vi "Initialize Device.vi"(8 "error in (no error)":errorcluster, 10 "VISA resource name":refnum<visa-resource-name>="COM9", 11 "Simulated in":refnum<class "Simulated.lvclass">) -> (0 "error out":errorcluster, 3 "Simulated out":refnum<class "Simulated.lvclass">)   [LabVIEW 2019, in "Simulated.lvclass"]
uses:
  Simulated.lvclass
  Abstract Spectrometer_class/Abstract Spectrometer.lvclass
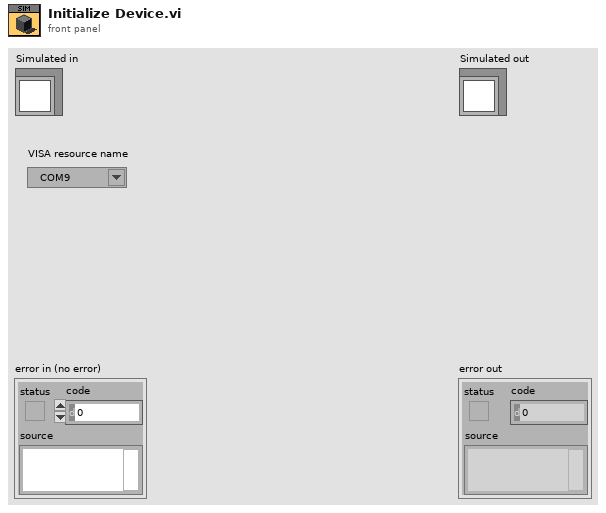
[diagram p1: front panel]
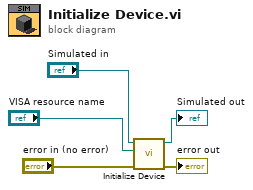
[diagram p0: block diagram]
diagram:
  n1 = call-parent "Initialize Device.vi"("error in (no error)"="error in (no error)", "VISA resource name"="VISA resource name", "Abstract Spectrometer in"="Simulated in") -> ("error out"=→"error out":errorcluster, "Abstract Spectrometer out"=→"Simulated out":refnum<class "Simulated.lvclass">)  [unwired: 7 in]
